vi "Y3(t).vi"(1 "Initial Position":dbl, 2 "L":dbl, 3 "W":dbl, 4 "V":dbl, 5 "T":dbl) -> (0 "Y3(t)":dbl)   [LabVIEW 2012]
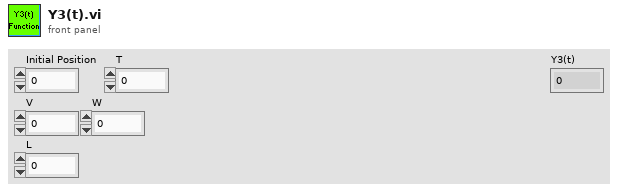
[diagram p1: front panel]
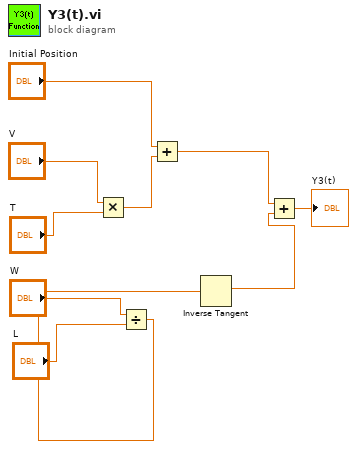
[diagram p0: block diagram]
diagram:
  n1 = Multiply(x="V", y="T") -> (x*y=w8:dbl)
  n2 = Divide(x="W", y="L") -> (x/y=w4:dbl)
  n3 = Add(x="Initial Position", y=w8) -> (x+y=w3:dbl)
  n4 = Inverse Tangent(1:w4) -> (0:w1:dbl)
  n5 = Add(x=w3, y=w1) -> (x+y=→"Y3(t)":dbl)
